vi "Tree Mouse Down.vi"(6 "PlatMods":T1, 8 "error in (no error)":errorcluster, 9 "Button":u16, 10 "Coords":cluster{"Horizontal":i32, "Vertical":i32}, 11 "Steps_Tree in":refnum<class "UI_Tree.lvclass">) -> (0 "error out":errorcluster, 3 "Steps_Tree out":refnum<class "UI_Tree.lvclass">)   [LabVIEW 2021, in "UI_Tree.lvlib" / "UI_Tree.lvclass"]
uses:
  UI_Tree.lvclass
  UI_Tree.lvclass/UI_Tree.ctl
  <userlib>/John_Lib/AbstractActorTemplate/AbstractActorTemplate/UIActorTop.lvclass
  C:/Program Files (x86)/National Instruments/LabVIEW 2021/user.lib/John_Lib/AbstractActorTemplate/AbstractActorTemplate/UIActorTop.lvclass
  C:/Program Files (x86)/National Instruments/LabVIEW 2021/vi.lib/ActorFramework/Actor/Actor.lvclass
  C:/Program Files (x86)/National Instruments/LabVIEW 2021/project/Create Actor from Template/_UI_Tree/UI_Tree.lvclass
panel:
  out "Active Cell:String":string
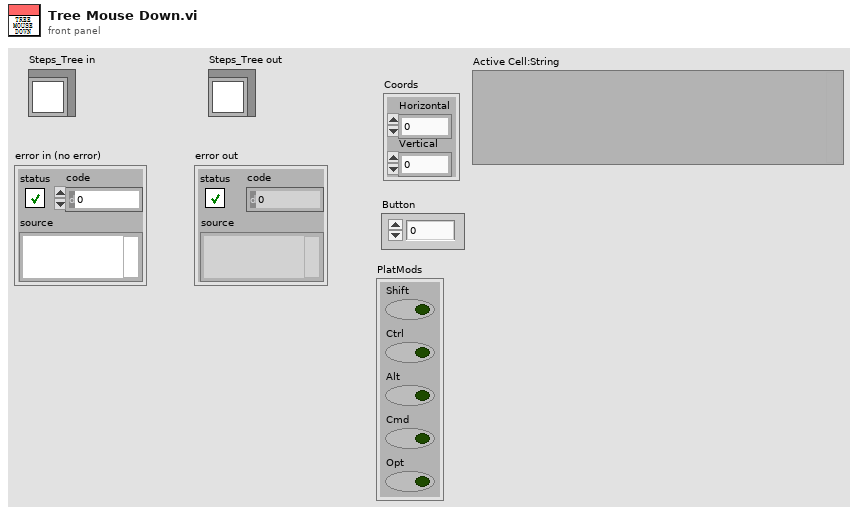
[diagram p1: front panel]
types:
  T1 = cluster{"Shift":bool, "Ctrl":bool, "Alt":bool, "Cmd":bool, "Opt":bool}
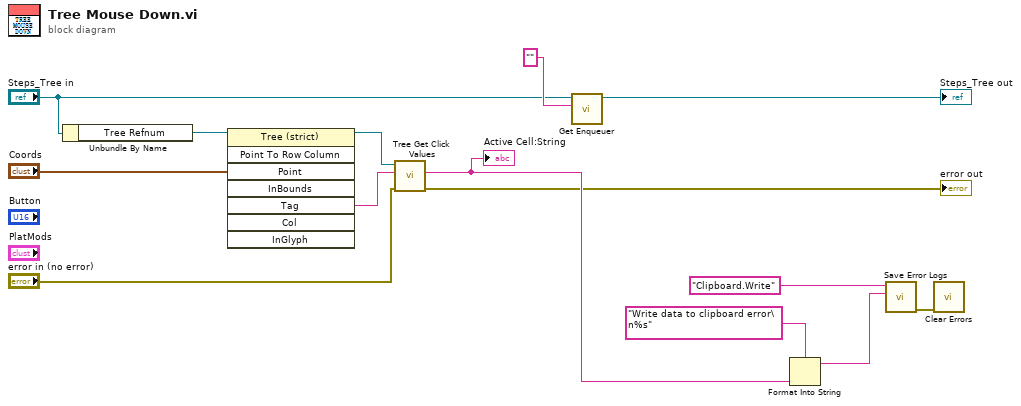
[diagram p0: block diagram]
diagram:
  n1 = Unbundle By Name("Steps_Tree in") -> ("Tree Refnum"=w13:refnum<vi>)
  n2 = invoke class="Tree (strict)" method="Point To Row Column"(reference=w13, "Point"="Coords") -> (reference out=w12:refnum<vi>, "Tag"=w11:string)  [unwired: 6 in, 6 out]
  n3 = call <userlib>:"Tree Get Click Values.vi"("error in (no error)"="error in (no error)", "Click Tag"=w11, "Tree Refnum"=w12) -> ("error out"=→"error out":errorcluster, "Active Cell:String"=w5:string)  [unwired: 5 in, 2 out]
  "Active Cell:String" <- w5
  n4 = call <userlib>:"Get Enqueuer.vi"("ActorQName"="", "UIActorTop in"="Steps_Tree in") -> ("UIActorTop out"=→"Steps_Tree out":refnum<class "UI_Tree.lvclass">)  [unwired: 3 in, 6 out]
  n5 = Format Into String(format string="Write data to clipboard error\n%s", w5) -> (resulting string=w4:string)  [unwired: 2 in, 1 out]
  n6 = call <userlib>:"Save Error Logs.vi"("States In"=w4, "FileName"="Clipboard.Write") -> ("error out"=w3:errorcluster)  [unwired: 9 in]
  n7 = call <vilib>:"Clear Errors.vi"("error in (no error)"=w3) -> ()  [unwired: 5 in, 2 out]
